vi "srv_tcpstr2data.vi"(10 "string":string[](array[string]), 11 "tags":string) -> (3 "values":dbl[][](array[numeric]))   [LabVIEW 2013]
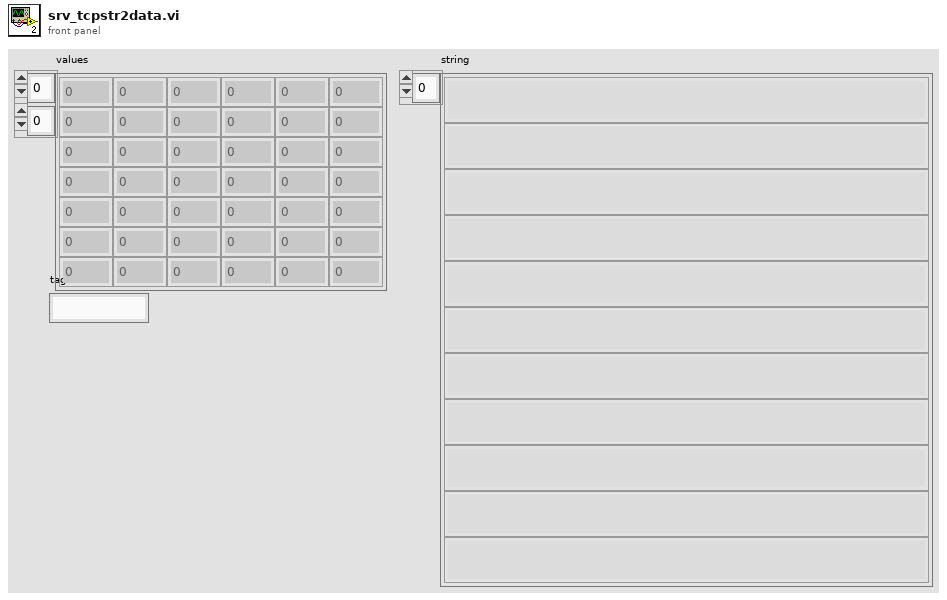
[diagram p1: front panel]
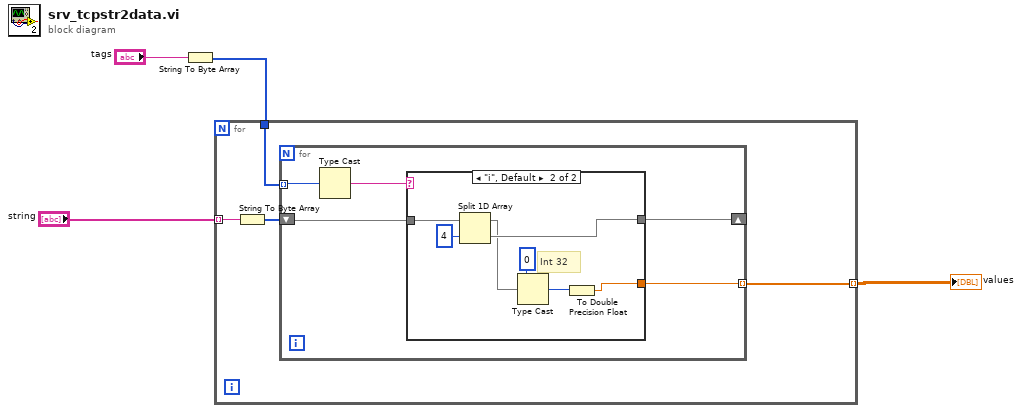
[diagram p0: block diagram]
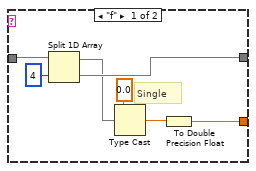
[diagram p2: hidden frame]
diagram:
  n1 = String To Byte Array(string="tags") -> (unsigned byte array=w3:u8[])
  n2 = for {
    tunnel: "string" -> [w6] mode=indexing
    tunnel: w3 -> [w8]
    tunnel: [w7] -> w1 mode=indexing
    n3 = String To Byte Array(string=w6) -> (unsigned byte array=w5:u8[])
    n4 = for {
      tunnel: w8 -> [w13] mode=indexing
      tunnel: [w11] -> w7 mode=indexing
      shift-right: [w9] -> _
      shift-left: w5 -> [w10]
      n5 = Type Cast(x=w13) -> (*(type *) &x=w12:string)  [unwired: 1 in]
      n6 = case shown="\"i\", Default" w12 {
        tunnel: [w14 w22] -> w11
        tunnel: w10 -> [w16 w27]
        tunnel: [w19 w25] -> w9
        frame "f" {
          # "Single"
          n7 = Split 1D Array(array=w16, index=4) -> (first subarray=w18:u8[], second subarray=w19:u8[])
          n8 = Type Cast(type=sgl 0.0, x=w18) -> (*(type *) &x=w15:sgl)
          n9 = To Double Precision Float(number=w15) -> (double precision float=w14:dbl)
        }
        frame "i", Default {
          # "Int 32"
          n10 = Split 1D Array(array=w27, index=4) -> (first subarray=w21:u8[], second subarray=w25:u8[])
          n11 = Type Cast(type=0, x=w21) -> (*(type *) &x=w23:i32)
          n12 = To Double Precision Float(number=w23) -> (double precision float=w22:dbl)
        }
      }
    }
  }
  "values" <- w1
